vi "check if paired.vi"(8 "error in":errorcluster, 11 "UDP Broadcast Editor Node in":refnum<class "TEC editor node.lvclass">) -> (0 "error out":errorcluster, 2 "paired":bool, 3 "UDP Broadcast Editor Node out":refnum<class "TEC editor node.lvclass">)   [LabVIEW 2013, in "TEC editor node.lvclass"]
uses:
  TEC editor node.lvclass
  read pair information.vi
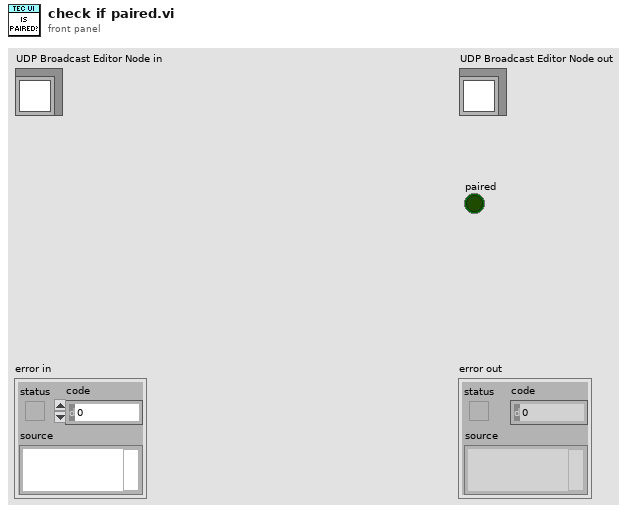
[diagram p1: front panel]
types:
  T1 = typedef "TEC editor node.lvclass/pair information.ctl" = cluster{"paired guid":string, "pair type":T2}
  T2 = typedef "TEC editor node.lvclass/pair type.ctl" = enum16{"master", "slave"}
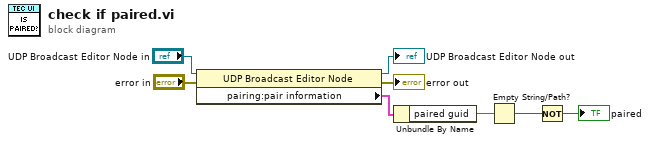
[diagram p0: block diagram]
diagram:
  n1 = property class="UDP Broadcast Editor Node"(reference="UDP Broadcast Editor Node in", error in="error in") -> (reference out=→"UDP Broadcast Editor Node out":refnum<class "TEC editor node.lvclass">, error out=→"error out":errorcluster, "pairing:pair information"=w4:T1)
  n2 = Unbundle By Name(w4) -> ("paired guid"=w3:string)
  n3 = Empty String/Path?(string/path=w3) -> (empty?=w2:bool)
  n4 = Not(x=w2) -> (.not. x?=→"paired":bool)
